vi "Check If Pixels Belong In SectorV2.vi"() -> (3 "FIFO Timeout?":bool)   [LabVIEW 2013]
uses:
  Globals/Pixel Location Global.vi
  Globals/Accumulated Sector Intensity.vi
  Globals/Sector Parameter Global.vi
  <vilib>/rvi/Memory/Memory_Emulation/nirvimemoryFastEmulationFpgaImpl.vi
  <instcachedir>/0/nirvimemoryFastEmulationFpgaImpl_5FBAB50466BC4C939F684F8805638BFC.lvgen/nirvimemoryFastEmulationFpgaImpl_5FBAB50466BC4C939F684F8805638BFC_013.vi
  <vilib>/rvi/DataTransferAndStorage/Container/Common/niFpgaContainerGetUniqueNameForEmu.vi
  <vilib>/rvi/Memory/Memory_Emulation/nirvimemoryFastEmulation.vi
  <vilib>/rvi/Memory/Memory_Emulation/nirvimemoryEmulation.vi
  <vilib>/rvi/FIFO/Fifo_Resource/nirvififoEmulationReadFpgaImpl.vi
  <vilib>/rvi/FIFO/Fifo_Resource/nirvififoEmulationWriteFpgaImpl.vi
  <vilib>/rvi/DataTransferAndStorage/Container/XNode/niFpgaContainer.xnode
  <vilib>/rvi/FIFO/Fifo_Resource/nirvififoEmulationRead.vi
  <vilib>/rvi/FIFO/Fifo_Resource/nirvififoEmulationWrite.vi
panel:
  out "End of  Data?":bool
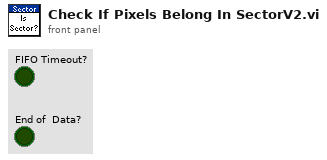
[diagram p1: front panel]
types:
  T1 = cluster{"Pixel Value":u8, "X":fxp<+,11,11>, "Y":fxp<+,11,11>}
  T2 = typedef "Sector Parameter Cluster.ctl" = cluster{"Start Angle":fxp<+/-,17,2>, "End Angle":fxp<+/-,17,2>, "Inner Radius":u16, "Outter Radius":u16, "Hinge X":u16, "Hinge Y":u16, "NumWingSectors":u8}
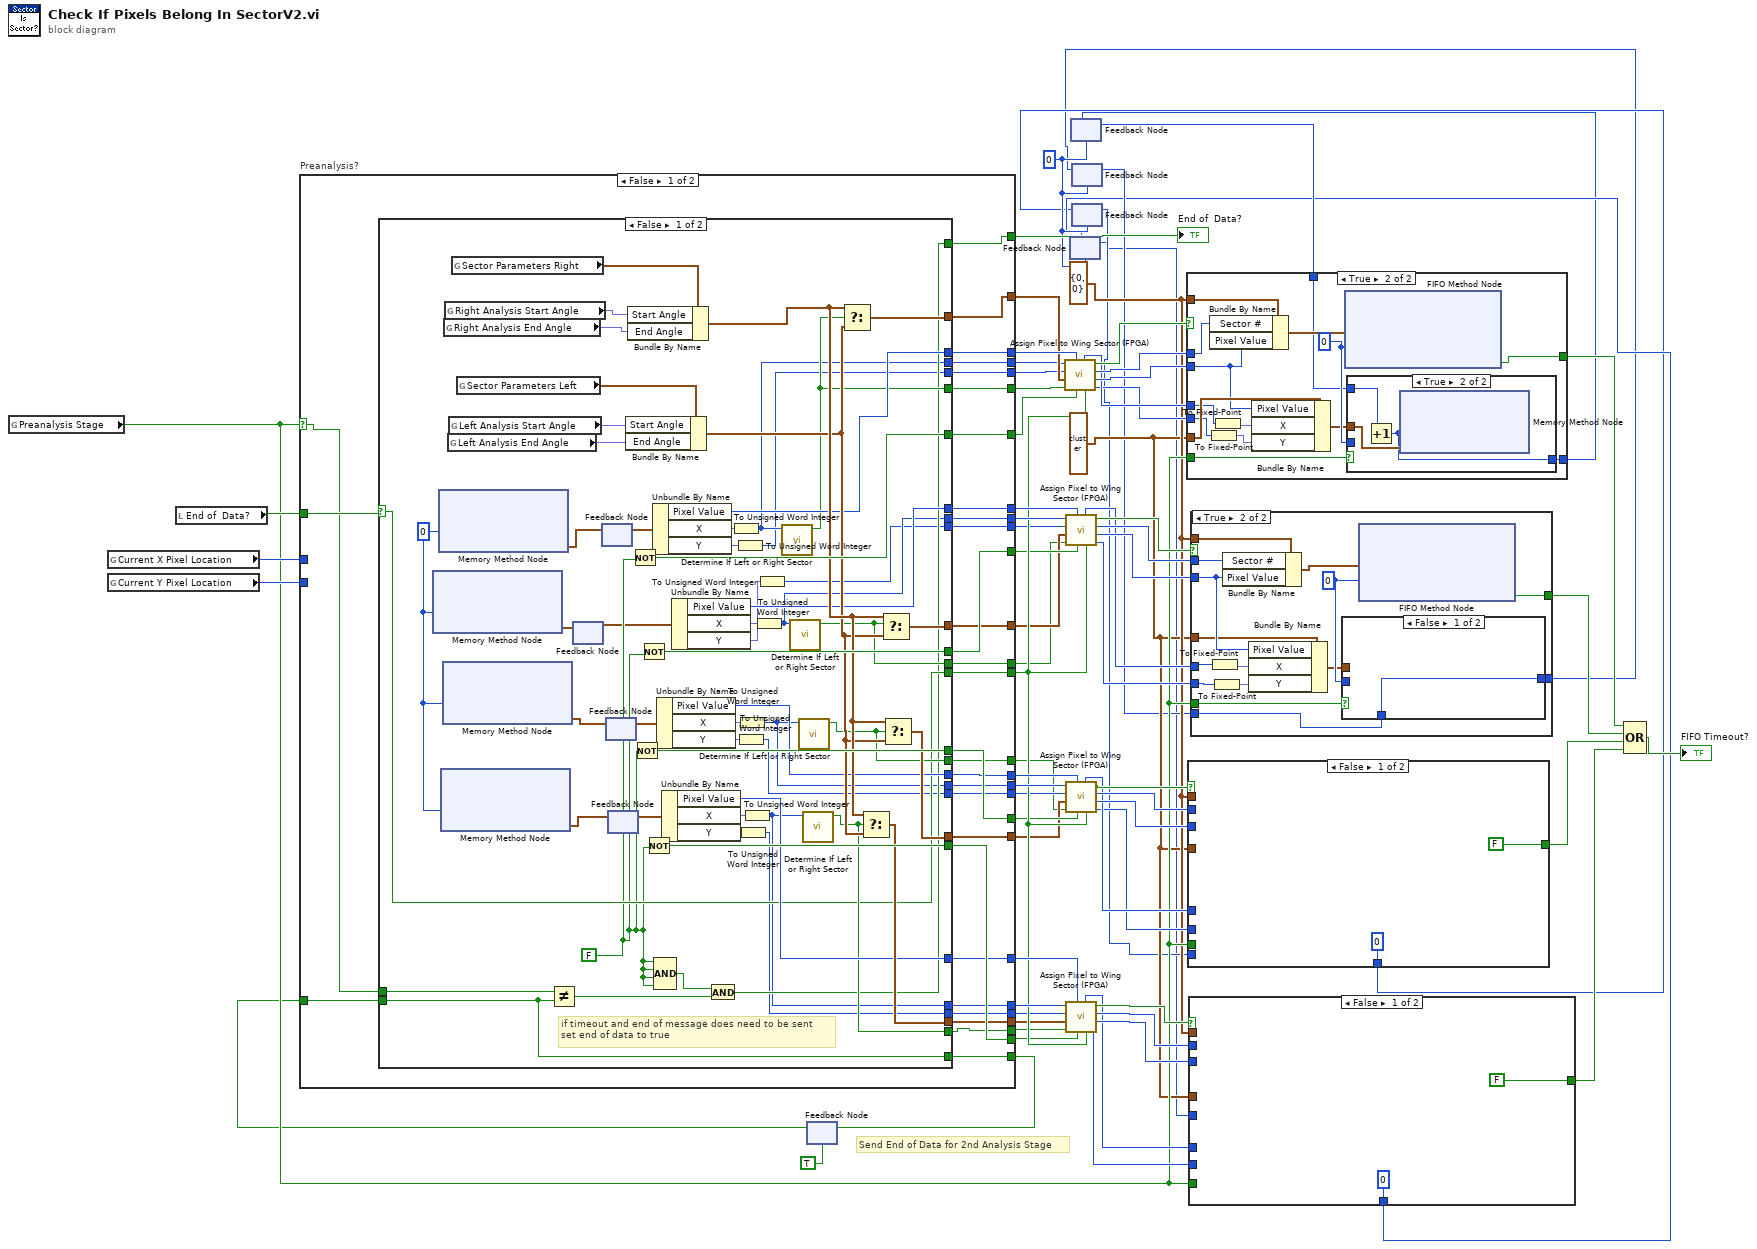
[diagram p0: block diagram]
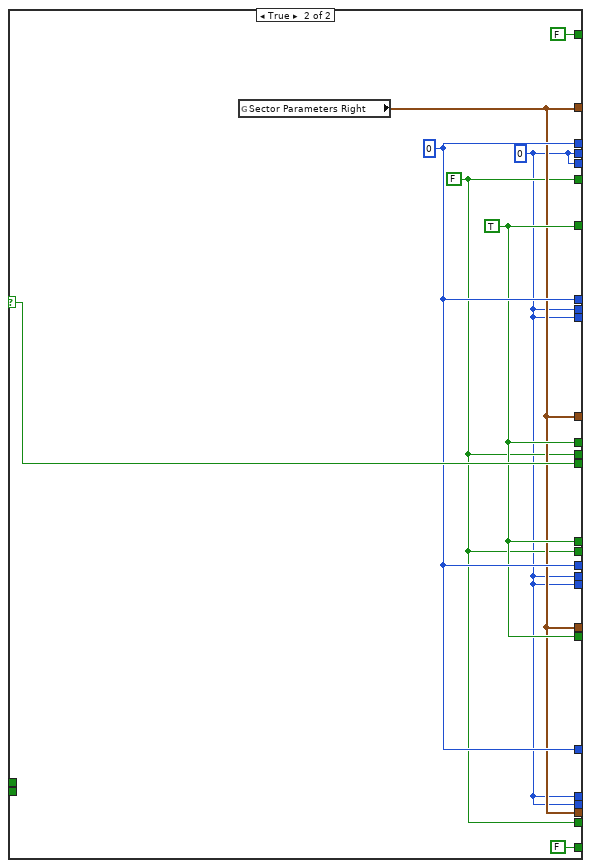
[diagram p2: hidden frame]
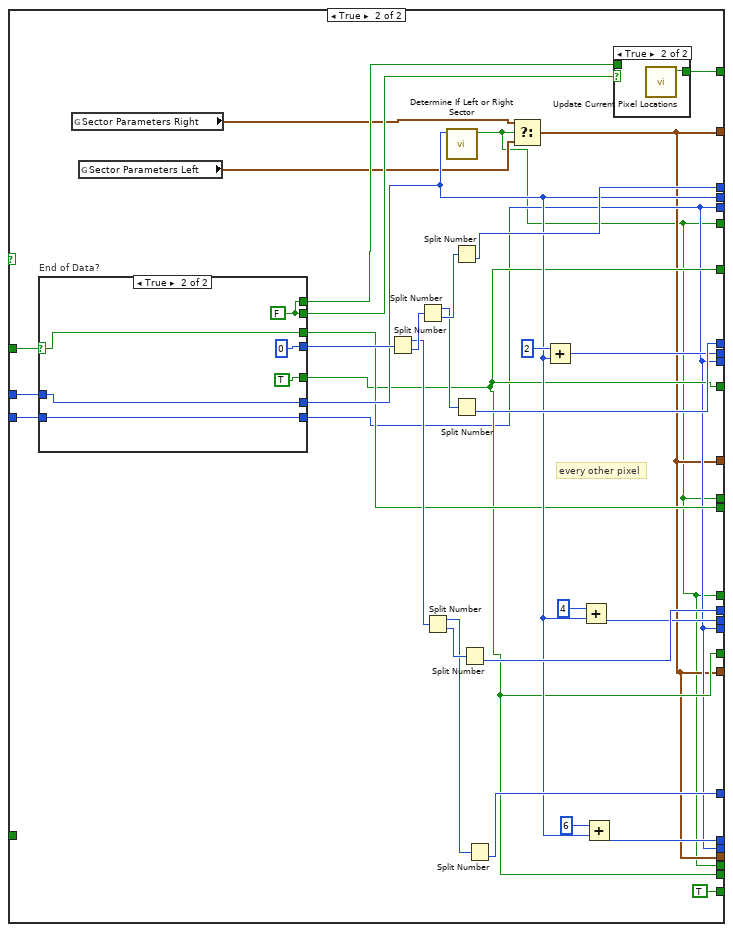
[diagram p3: hidden frame]
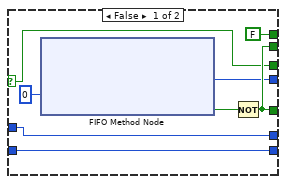
[diagram p4: hidden frame]
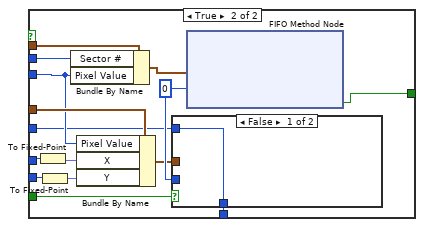
[diagram p6: hidden frame]
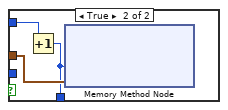
[diagram p7: hidden frame]
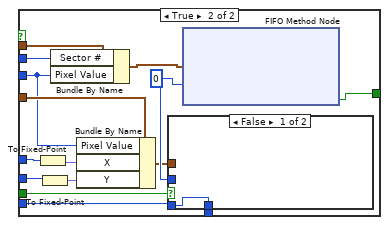
[diagram p8: hidden frame]
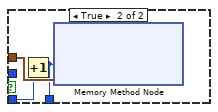
[diagram p9: hidden frame]
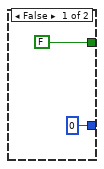
[diagram p10: hidden frame]
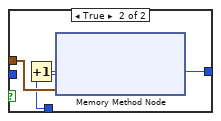
[diagram p11: hidden frame]
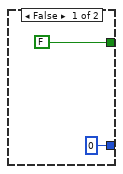
[diagram p12: hidden frame]
diagram:
  w5 = u32 0 ("Address")
  w10 = T1 {"Pixel Value"=0, "X"=0.0, "Y"=0.0} ("Element")
  w11 = cluster{"Sector #":u8, "Pixel Value":u8} {"Sector #"=0, "Pixel Value"=0} ("Element")
  # "Send End of Data for 2nd Analysis Stage"
  n1 = global read "Accumulated Sector Intensity.vi" "Preanalysis Stage"() -> (w27:bool)
  n2 = global read "Pixel Location Global.vi" "Current X Pixel Location"() -> (w38:u16)
  n3 = global read "Pixel Location Global.vi" "Current Y Pixel Location"() -> (w40:u16)
  n4 = local read "End of  Data?"() -> (w42:bool)
  n5 = feedback #1(TRUE) -> (w13:bool)
  n6 = case "Preanalysis?" shown="False" w27 {
    selector: w27 -> [w71 _]
    tunnel: [w94 w195] -> w69
    tunnel: [w76 w165] -> w51
    tunnel: [w88 w187] -> w50
    tunnel: [w87 w186] -> w49
    tunnel: [w86 w185] -> w48
    tunnel: [w85 w184] -> w47
    tunnel: [w83 w180] -> w46
    tunnel: [w82 w179] -> w45
    tunnel: [w81 w178] -> w44
    tunnel: [w92 w166] -> w43
    tunnel: [w98 w168] -> w28
    tunnel: w42 -> [w99 w175]
    tunnel: [w80 w167] -> w41
    tunnel: w40 -> [_ w174]
    tunnel: [w84 w173] -> w39
    tunnel: w38 -> [_ w172]
    tunnel: [w93 w171] -> w37
    tunnel: [w97 w168] -> w26
    tunnel: [w96 w168] -> w25
    tunnel: [w95 w168] -> w24
    tunnel: [w91 w166] -> w23
    tunnel: [w90 w166] -> w22
    tunnel: [w89 w166] -> w21
    tunnel: [w79 w167] -> w20
    tunnel: [w78 w167] -> w19
    tunnel: [w77 w167] -> w18
    tunnel: [w75 w165] -> w17
    tunnel: [w74 w165] -> w16
    tunnel: [w73 w165] -> w15
    tunnel: w13 -> [w72 _]
    tunnel: [w70 TRUE] -> w12
    frame False {
      n7 = case shown="False" w99 {
        selector: w99 -> [w123 w162]
        tunnel: [w149 w160] -> w98
        tunnel: [w148 w160] -> w97
        tunnel: [w147 w160] -> w96
        tunnel: [w146 w160] -> w95
        tunnel: [w119 FALSE] -> w94
        tunnel: [w123 w162] -> w93
        tunnel: [w145 w159] -> w92
        tunnel: [w144 w159] -> w91
        tunnel: [w143 w159] -> w90
        tunnel: [w140 w159] -> w89
        tunnel: [w139 w161] -> w88
        tunnel: [w138 w161] -> w87
        tunnel: [w137 w161] -> w86
        tunnel: [w136 w161] -> w85
        tunnel: [w117 w157] -> w84
        tunnel: [w115 w157] -> w83
        tunnel: [w113 w157] -> w82
        tunnel: [w111 w157] -> w81
        tunnel: [w116 w157] -> w80
        tunnel: [w114 w157] -> w79
        tunnel: [w112 w157] -> w78
        tunnel: [w110 w157] -> w77
        tunnel: [w127 w158] -> w76
        tunnel: [w126 w158] -> w75
        tunnel: [w125 w158] -> w74
        tunnel: [w124 w158] -> w73
        tunnel: w72 -> [w118 _]
        tunnel: w71 -> [w122 _]
        tunnel: [w118 FALSE] -> w70
        frame False {
          w104 = u32 0 ("Address")
          w105 = FALSE ("x")
          # "if timeout and end of message does need to be sent\nset end of data to true"
          n8 = xnode ("Memory Method Node")("Address"=w104) -> ("Data"=w108:T1)  [unwired: 1 in, 1 out]
          n9 = xnode ("Memory Method Node")("Address"=w104) -> ("Data"=w109:T1)  [unwired: 1 in, 1 out]
          n10 = xnode ("Memory Method Node")("Address"=w104) -> ("Data"=w106:T1)  [unwired: 1 in, 1 out]
          n11 = xnode ("Memory Method Node")("Address"=w104) -> ("Data"=w107:T1)  [unwired: 1 in, 1 out]
          n12 = global read "Sector Parameter Global.vi" "Right Analysis End Angle"() -> (w153:fxp<+/-,17,2>)
          n13 = global read "Sector Parameter Global.vi" "Right Analysis Start Angle"() -> (w154:fxp<+/-,17,2>)
          n14 = global read "Sector Parameter Global.vi" "Left Analysis End Angle"() -> (w150:fxp<+/-,17,2>)
          n15 = global read "Sector Parameter Global.vi" "Left Analysis Start Angle"() -> (w151:fxp<+/-,17,2>)
          n16 = global read "Sector Parameter Global.vi" "Sector Parameters Right"() -> (w155:T2)
          n17 = global read "Sector Parameter Global.vi" "Sector Parameters Left"() -> (w152:T2)
          n18 = Not Equal?(x=w122, y=w118) -> (x != y?=w120:bool)
          n19 = feedback-in #2(w108) -> ()
          n20 = feedback #2() -> (w102:T1)  [unwired: 1 in]
          n21 = feedback-in #3(w109) -> ()
          n22 = feedback #3() -> (w103:T1)  [unwired: 1 in]
          n23 = feedback-in #4(w107) -> ()
          n24 = feedback #4() -> (w101:T1)  [unwired: 1 in]
          n25 = feedback-in #5(w106) -> ()
          n26 = feedback #5() -> (w100:T1)  [unwired: 1 in]
          n27 = Bundle By Name(cluster=w152, "Start Angle"=w151, "End Angle"=w150) -> (w141:T2)
          n28 = Bundle By Name(cluster=w155, "Start Angle"=w154, "End Angle"=w153) -> (w142:T2)
          n29 = Not(x=w105) -> (.not. x?=w146:bool)
          n30 = Not(x=w105) -> (.not. x?=w148:bool)
          n31 = Not(x=w105) -> (.not. x?=w147:bool)
          n32 = Not(x=w105) -> (.not. x?=w149:bool)
          n33 = Unbundle By Name(w103) -> ("Pixel Value"=w139:u8, "X"=w135:fxp<+,11,11>, "Y"=w131:fxp<+,11,11>)
          n34 = Compound Arithmetic op=AND(w105, w105, w105, w105) -> (w121:bool)
          n35 = Unbundle By Name(w101) -> ("Pixel Value"=w137:u8, "X"=w133:fxp<+,11,11>, "Y"=w129:fxp<+,11,11>)
          n36 = Unbundle By Name(w100) -> ("Pixel Value"=w136:u8, "X"=w132:fxp<+,11,11>, "Y"=w128:fxp<+,11,11>)
          n37 = Unbundle By Name(w102) -> ("Pixel Value"=w138:u8, "X"=w134:fxp<+,11,11>, "Y"=w130:fxp<+,11,11>)
          n38 = And(x=w121, y=w120) -> (x .and. y?=w119:bool)
          n39 = To Unsigned Word Integer(number=w135) -> (unsigned 16bit integer=w117:u16)
          n40 = To Unsigned Word Integer(number=w131) -> (unsigned 16bit integer=w116:u16)
          n41 = To Unsigned Word Integer(number=w129) -> (unsigned 16bit integer=w112:u16)
          n42 = To Unsigned Word Integer(number=w133) -> (unsigned 16bit integer=w113:u16)
          n43 = To Unsigned Word Integer(number=w128) -> (unsigned 16bit integer=w110:u16)
          n44 = To Unsigned Word Integer(number=w132) -> (unsigned 16bit integer=w111:u16)
          n45 = To Unsigned Word Integer(number=w134) -> (unsigned 16bit integer=w115:u16)
          n46 = To Unsigned Word Integer(number=w130) -> (unsigned 16bit integer=w114:u16)
          n47 = call "Determine If Left or Right Sector.vi"("X Pixel Location"=w117) -> ("Right Sector?"=w127:bool)  [unwired: 10 in]
          n48 = call "Determine If Left or Right Sector.vi"("X Pixel Location"=w115) -> ("Right Sector?"=w126:bool)  [unwired: 10 in]
          n49 = call "Determine If Left or Right Sector.vi"("X Pixel Location"=w113) -> ("Right Sector?"=w125:bool)  [unwired: 10 in]
          n50 = call "Determine If Left or Right Sector.vi"("X Pixel Location"=w111) -> ("Right Sector?"=w124:bool)  [unwired: 10 in]
          n51 = Select(t=w142, s=w127, f=w141) -> (s? t:f=w145:T2)
          n52 = Select(t=w142, s=w124, f=w141) -> (s? t:f=w140:T2)
          n53 = Select(t=w142, s=w126, f=w141) -> (s? t:f=w144:T2)
          n54 = Select(t=w142, s=w125, f=w141) -> (s? t:f=w143:T2)
        }
        frame True {
          w157 = u16 0 ("X")
          w158 = FALSE ("Right Sector?")
          w160 = TRUE
          w161 = u8 0 ("Pixel Value")
          n55 = global read "Sector Parameter Global.vi" "Sector Parameters Right"() -> (w159:T2)
        }
      }
    }
    frame True {
      # "every other pixel"
      n56 = case "End of Data?" shown="True" w175 {
        selector: w175 -> [w197 w204]
        tunnel: [w201 TRUE ("Timed Out?")] -> w168
        tunnel: [w196 u64 0 ("Element")] -> w194
        tunnel: [w201 w207] -> w177
        tunnel: [FALSE ("Timed Out?") w207] -> w176
        tunnel: [w199 w205] -> w167
        tunnel: w174 -> [w199 w205]
        tunnel: [w198 w206] -> w173
        tunnel: w172 -> [w198 w206]
        tunnel: [w197 w204] -> w171
        frame False {
          n57 = xnode ("FIFO Method Node")("Timeout"=0) -> ("Element"=w196:u64, "Timed Out?"=w202:bool)  [unwired: 1 in, 1 out]
          n58 = Not(x=w202) -> (.not. x?=w201:bool)
        }
        frame True {
          w207 = FALSE ("Timed Out?")
        }
      }
      n59 = global read "Sector Parameter Global.vi" "Sector Parameters Right"() -> (w170:T2)
      n60 = global read "Sector Parameter Global.vi" "Sector Parameters Left"() -> (w169:T2)
      n61 = Split Number(x=w194) -> (hi(x)=w192:u32, lo(x)=w193:u32)
      n62 = Split Number(x=w193) -> (hi(x)=w190:u16, lo(x)=w191:u16)
      n63 = Split Number(x=w192) -> (hi(x)=w188:u16, lo(x)=w189:u16)
      n64 = call "Determine If Left or Right Sector.vi"("X Pixel Location"=w173) -> ("Right Sector?"=w165:bool)  [unwired: 10 in]
      n65 = Split Number(x=w191) -> (lo(x)=w187:u8)  [unwired: 1 out]
      n66 = Split Number(x=w190) -> (lo(x)=w186:u8)  [unwired: 1 out]
      n67 = Split Number(x=w189) -> (lo(x)=w185:u8)  [unwired: 1 out]
      n68 = Split Number(x=w188) -> (lo(x)=w184:u8)  [unwired: 1 out]
      n69 = Select(t=w170, s=w165, f=w169) -> (s? t:f=w166:T2)
      n70 = Add(x=u16 2, y=w173) -> (x+y=w180:u16)
      n71 = Add(x=u16 4, y=w173) -> (x+y=w179:u16)
      n72 = Add(x=u16 6, y=w173) -> (x+y=w178:u16)
      n73 = case shown="True" w177 {
        tunnel: [w210 w211] -> w195
        tunnel: w176 -> [w210 _]
        frame False {
        }
        frame True {
          n74 = call "Update Current Pixel Locations.vi"() -> ("End of data?"=w211:bool)  [unwired: 11 in]
        }
      }
    }
  }
  "End of  Data?" <- w69
  n75 = feedback-in #1(w12) -> ()
  n76 = call "Assign Pixel to Wing Sector (FPGA).vi"("End of Data?"=w37, "Valid Data?"=w24, "Pixel Intensity In"=w50, "Right Wing?"=w51, "Sector Parameters"=w43, "Pixel Y"=w41, "Pixel X"=w39) -> ("Y"=w35:u16, "Pixel Intensity Out"=w61:u8, "sector #"=w62:u8, "output valid"=w63:bool, "X"=w36:u16)
  n77 = call "Assign Pixel to Wing Sector (FPGA).vi"("End of Data?"=w37, "Valid Data?"=w25, "Pixel Intensity In"=w49, "Right Wing?"=w17, "Sector Parameters"=w23, "Pixel Y"=w20, "Pixel X"=w46) -> ("Y"=w33:u16, "Pixel Intensity Out"=w58:u8, "sector #"=w59:u8, "output valid"=w60:bool, "X"=w34:u16)
  n78 = call "Assign Pixel to Wing Sector (FPGA).vi"("End of Data?"=w37, "Valid Data?"=w26, "Pixel Intensity In"=w48, "Right Wing?"=w16, "Sector Parameters"=w22, "Pixel Y"=w19, "Pixel X"=w45) -> ("Y"=w31:u16, "Pixel Intensity Out"=w55:u8, "sector #"=w56:u8, "output valid"=w57:bool, "X"=w32:u16)
  n79 = call "Assign Pixel to Wing Sector (FPGA).vi"("End of Data?"=w37, "Valid Data?"=w28, "Pixel Intensity In"=w47, "Right Wing?"=w15, "Sector Parameters"=w21, "Pixel Y"=w18, "Pixel X"=w44) -> ("Y"=w29:u16, "Pixel Intensity Out"=w52:u8, "sector #"=w53:u8, "output valid"=w54:bool, "X"=w30:u16)
  n80 = feedback #6(w5) -> (w6:u32)
  n81 = feedback #7(w5) -> (w9:u32)
  n82 = feedback #8(w5) -> (w8:u32)
  n83 = feedback #9(w5) -> (w7:u32)
  n84 = case shown="True" w63 {
    tunnel: w11 -> [_ w225]
    tunnel: [FALSE ("Timed Out?") w227] -> w67
    tunnel: w62 -> [_ w224]
    tunnel: w61 -> [_ w222]
    tunnel: w36 -> [_ w220]
    tunnel: w35 -> [_ w218]
    tunnel: w27 -> [_ w226]
    tunnel: w10 -> [_ w223]
    tunnel: w9 -> [_ w215]
    tunnel: [u32 0 ("Address") w214] -> w1
    frame False {
    }
    frame True {
      w228 = 0 ("Timeout")
      n85 = To Fixed-Point(number=w218) -> (fixed-point=w217:fxp<+,11,11>)  [unwired: 1 in]
      n86 = Bundle By Name(cluster=w225, "Sector #"=w224, "Pixel Value"=w222) -> (w216:cluster{"Sector #":u8, "Pixel Value":u8})
      n87 = To Fixed-Point(number=w220) -> (fixed-point=w219:fxp<+,11,11>)  [unwired: 1 in]
      n88 = Bundle By Name(cluster=w223, "Pixel Value"=w222, "X"=w219, "Y"=w217) -> (w221:T1)
      n89 = xnode ("FIFO Method Node")("Element"=w216, "Timeout"=w228) -> ("Timed Out?"=w227:bool)  [unwired: 1 in, 1 out]
      n90 = case shown="True" w226 {
        tunnel: w228 -> [_ _]
        tunnel: w221 -> [_ w231]
        tunnel: w215 -> [w229 w232]
        tunnel: [w229 w230] -> w214
        frame False {
        }
        frame True {
          n91 = Increment(x=w232) -> (x+1=w230:u32)
          n92 = xnode ("Memory Method Node")("Address"=w230, "Data"=w231) -> ()  [unwired: 1 in, 1 out]
        }
      }
    }
  }
  n93 = feedback-in #7(w1) -> ()
  n94 = case shown="False" w57 {
    tunnel: w11 -> [_ w247]
    tunnel: [FALSE ("Timed Out?") w249] -> w65
    tunnel: w56 -> [_ w246]
    tunnel: w55 -> [_ w238]
    tunnel: w32 -> [_ w240]
    tunnel: w31 -> [_ w239]
    tunnel: w27 -> [_ w245]
    tunnel: w10 -> [_ w242]
    tunnel: w7 -> [_ w236]
    tunnel: [u32 0 ("Address") w235] -> w3
    frame False {
    }
    frame True {
      w248 = 0 ("Timeout")
      n95 = To Fixed-Point(number=w240) -> (fixed-point=w244:fxp<+,11,11>)  [unwired: 1 in]
      n96 = To Fixed-Point(number=w239) -> (fixed-point=w243:fxp<+,11,11>)  [unwired: 1 in]
      n97 = Bundle By Name(cluster=w247, "Sector #"=w246, "Pixel Value"=w238) -> (w237:cluster{"Sector #":u8, "Pixel Value":u8})
      n98 = Bundle By Name(cluster=w242, "Pixel Value"=w238, "X"=w244, "Y"=w243) -> (w241:T1)
      n99 = case shown="False" w245 {
        tunnel: w248 -> [_ _]
        tunnel: w241 -> [_ w253]
        tunnel: w236 -> [w250 w252]
        tunnel: [w250 w251] -> w235
        frame False {
        }
        frame True {
          n100 = Increment(x=w252) -> (x+1=w251:u32)
          n101 = xnode ("Memory Method Node")("Address"=w251, "Data"=w253) -> ()  [unwired: 1 in, 1 out]
        }
      }
      n102 = xnode ("FIFO Method Node")("Element"=w237, "Timeout"=w248) -> ("Timed Out?"=w249:bool)  [unwired: 1 in, 1 out]
    }
  }
  n103 = feedback-in #9(w3) -> ()
  n104 = case shown="False" w54 {
    tunnel: w11 -> [_ w268]
    tunnel: [FALSE ("Timed Out?") w269] -> w64
    tunnel: w53 -> [_ w267]
    tunnel: w52 -> [_ w262]
    tunnel: w30 -> [_ w261]
    tunnel: w29 -> [_ w260]
    tunnel: w27 -> [_ w266]
    tunnel: w10 -> [_ w263]
    tunnel: w6 -> [_ w257]
    tunnel: [u32 0 ("Address") w256] -> w4
    frame False {
    }
    frame True {
      w270 = 0 ("Timeout")
      n105 = To Fixed-Point(number=w261) -> (fixed-point=w264:fxp<+,11,11>)  [unwired: 1 in]
      n106 = To Fixed-Point(number=w260) -> (fixed-point=w265:fxp<+,11,11>)  [unwired: 1 in]
      n107 = Bundle By Name(cluster=w268, "Sector #"=w267, "Pixel Value"=w262) -> (w258:cluster{"Sector #":u8, "Pixel Value":u8})
      n108 = Bundle By Name(cluster=w263, "Pixel Value"=w262, "X"=w264, "Y"=w265) -> (w259:T1)
      n109 = case shown="False" w266 {
        tunnel: w270 -> [_ _]
        tunnel: w259 -> [_ w274]
        tunnel: w257 -> [w271 w273]
        tunnel: [w271 w272] -> w256
        frame False {
        }
        frame True {
          n110 = Increment(x=w273) -> (x+1=w272:u32)
          n111 = xnode ("Memory Method Node")("Address"=w272, "Data"=w274) -> ()  [unwired: 1 in, 1 out]
        }
      }
      n112 = xnode ("FIFO Method Node")("Element"=w258, "Timeout"=w270) -> ("Timed Out?"=w269:bool)  [unwired: 1 in, 1 out]
    }
  }
  n113 = feedback-in #6(w4) -> ()
  n114 = case shown="True" w60 {
    tunnel: w11 -> [_ w289]
    tunnel: [FALSE ("Timed Out?") w290] -> w66
    tunnel: w59 -> [_ w288]
    tunnel: w58 -> [_ w284]
    tunnel: w34 -> [_ w282]
    tunnel: w33 -> [_ w283]
    tunnel: w27 -> [_ w287]
    tunnel: w10 -> [_ w281]
    tunnel: w8 -> [_ w278]
    tunnel: [u32 0 ("Address") w277] -> w2
    frame False {
    }
    frame True {
      w291 = 0 ("Timeout")
      n115 = To Fixed-Point(number=w282) -> (fixed-point=w285:fxp<+,11,11>)  [unwired: 1 in]
      n116 = To Fixed-Point(number=w283) -> (fixed-point=w286:fxp<+,11,11>)  [unwired: 1 in]
      n117 = Bundle By Name(cluster=w289, "Sector #"=w288, "Pixel Value"=w284) -> (w279:cluster{"Sector #":u8, "Pixel Value":u8})
      n118 = Bundle By Name(cluster=w281, "Pixel Value"=w284, "X"=w285, "Y"=w286) -> (w280:T1)
      n119 = case shown="False" w287 {
        tunnel: w291 -> [_ _]
        tunnel: w280 -> [_ w295]
        tunnel: w278 -> [w292 w294]
        tunnel: [w292 w293] -> w277
        frame False {
        }
        frame True {
          n120 = Increment(x=w294) -> (x+1=w293:u32)
          n121 = xnode ("Memory Method Node")("Address"=w293, "Data"=w295) -> ()  [unwired: 1 in, 1 out]
        }
      }
      n122 = xnode ("FIFO Method Node")("Element"=w279, "Timeout"=w291) -> ("Timed Out?"=w290:bool)  [unwired: 1 in, 1 out]
    }
  }
  n123 = feedback-in #8(w2) -> ()
  n124 = Compound Arithmetic op=OR(w67, w66, w65, w64) -> (→"FIFO Timeout?":bool)
